vi "_Ping.vi"(0 "device name":string) -> (1 "success":bool, 2 "error code":i32)   [LabVIEW 2014, in "tango.lvlib"]
uses:
  tango.lvlib
  tango_binding.so
panel:
  out "error stack":string[](array[string])
  # "This Vi is deprecated and only maintained for backward compatibility. Please use  _TangoPing instead."
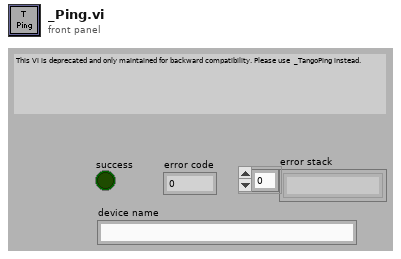
[diagram p1: front panel]
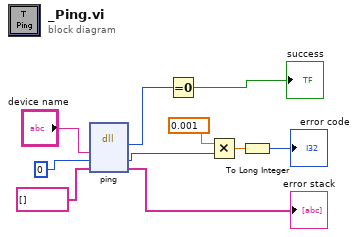
[diagram p0: block diagram]
diagram:
  n1 = dll-call lib="tango_binding.*" fn="ping"("dev_name"="device name", "rtt"=0, "error_stack"=string[] [] ("Error Stack")) -> ("return type"=w4:i32, "rtt"=w10:u32, "error_stack"=→"error stack":string[])  [unwired: 4 in, 2 out]
  n2 = Equal To 0?(x=w4) -> (x = 0?=→"success":bool)
  n3 = Multiply(x=0.001, y=w10) -> (x*y=w7:dbl)
  n4 = To Long Integer(number=w7) -> (32bit integer=→"error code":i32)
